vi "Untitled 5.vi"() -> ()   [LabVIEW 2020]
panel:
  in  "VISA resource name":refnum<visa-resource-name>
  in  "Table Control":string[][](table)
  out "Humidity Chart":i32(graph)
  out "Temperature Chart":i32(graph)
  out "Humidity":dbl(knob) scale=0.0..100.0
  out "Temperature":dbl(slide) scale=0.0..100.0
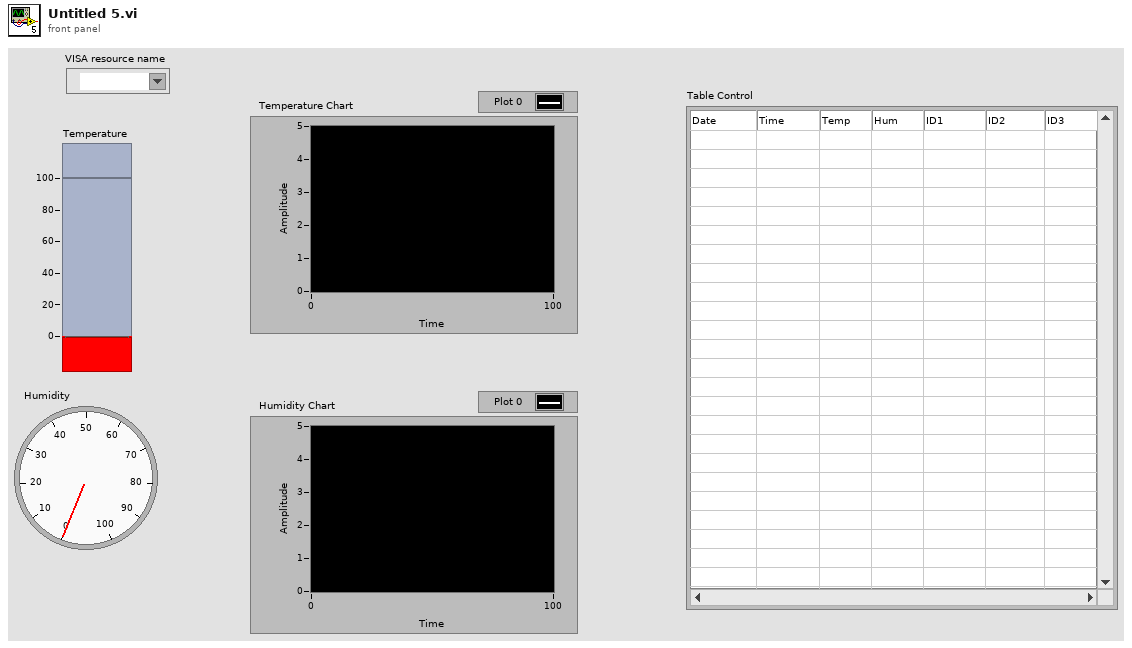
[diagram p1: front panel]
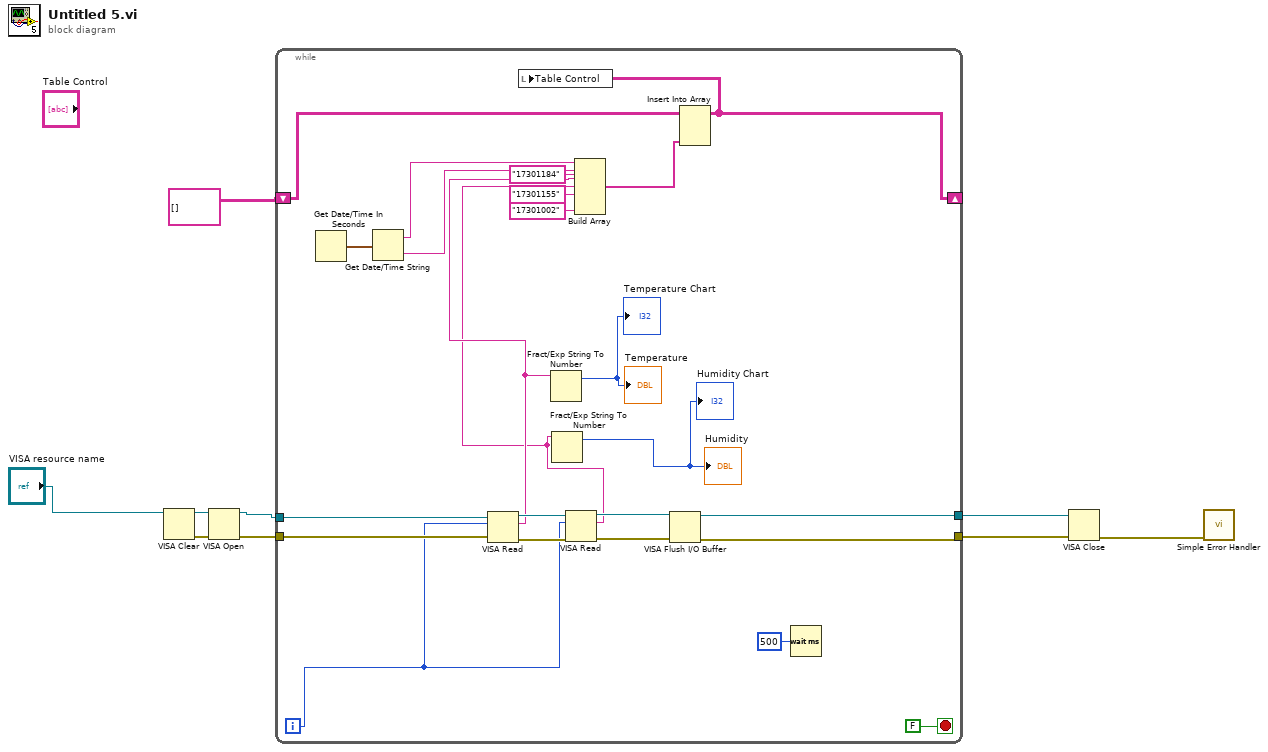
[diagram p0: block diagram]
diagram:
  n1 = VISA Clear(VISA resource name="VISA resource name") -> (VISA resource name out=w9:refnum<visa-resource-name>, error out=w8:errorcluster)  [unwired: 1 in]
  n2 = VISA Open(error in (no error)=w8, VISA resource name=w9) -> (VISA resource name=w7:refnum<visa-resource-name>, error out=w6:errorcluster)  [unwired: 3 in]
  n3 = while {
    tunnel: w7 -> [w33]
    tunnel: w6 -> [w32]
    tunnel: [w27] -> w5
    tunnel: [w26] -> w4
    shift-right: [w23] -> _
    shift-left: string[][] [] -> [w24]
    i -> [w20]
    stop <- FALSE stop-if-true
    n4 = Get Date/Time In Seconds() -> (seconds since 1Jan1904=w19:timestamp)
    n5 = Get Date/Time String(seconds (now)=w19) -> (date string=w18:string, time string=w17:string)  [unwired: 2 in]
    n6 = VISA Read(VISA resource name=w33, byte count=w20, error in (no error)=w32) -> (VISA resource name out=w31:refnum<visa-resource-name>, read buffer=w16:string, error out=w30:errorcluster)  [unwired: 1 out]
    n7 = Fract/Exp String To Number(string=w16) -> (offset past number=→"Temperature" →"Temperature Chart":i32)  [unwired: 3 in, 1 out]
    n8 = VISA Read(VISA resource name=w31, byte count=w20, error in (no error)=w30) -> (VISA resource name out=w29:refnum<visa-resource-name>, read buffer=w15:string, error out=w28:errorcluster)  [unwired: 1 out]
    n9 = Fract/Exp String To Number(string=w15) -> (offset past number=→"Humidity" →"Humidity Chart":i32)  [unwired: 3 in, 1 out]
    n10 = Build Array(w18, w17, w16, w15, "17301155" ("element"), "17301184" ("element"), "17301002" ("element")) -> (w11:string[])
    n11 = VISA Flush I/O Buffer(VISA resource name=w29, error in (no error)=w28) -> (VISA resource name out=w27:refnum<visa-resource-name>, error out=w26:errorcluster)  [unwired: 1 in]
    n12 = Insert Into Array(array=w24, new element=w11) -> (w23:string[][])  [unwired: 2 in]
    n13 = local write "Table Control"(w23) -> ()
    n14 = Wait (ms)(milliseconds to wait=u32 500) -> ()  [unwired: 1 out]
  }
  n15 = VISA Close(VISA resource name=w5, error in (no error)=w4) -> (error out=w3:errorcluster)
  n16 = call <vilib>:"Simple Error Handler.vi"("error in (no error)"=w3) -> ()  [unwired: 4 in, 5 out]
